vi "onHttpPatch (Buffer).vi"(8 "error in":errorcluster, 10 "httpRequest":refnum<class "httpRequest.lvclass">, 11 "http-method in":refnum<class "HttpClient.Basic.lvclass">) -> (0 "error out":errorcluster, 2 "httpResponse":refnum<class "httpResponse.lvclass">, 3 "http-method out":refnum<class "HttpClient.Basic.lvclass">)   [LabVIEW 2020, in "httpClient.lvlib" / "HttpClient.Basic.lvclass"]
uses:
  HttpClient.Basic.lvclass
  HttpClient.Basic.lvclass/HttpClient.Basic.ctl
  httpResponse/httpResponse.lvclass
  httpRequest/httpRequest.lvclass
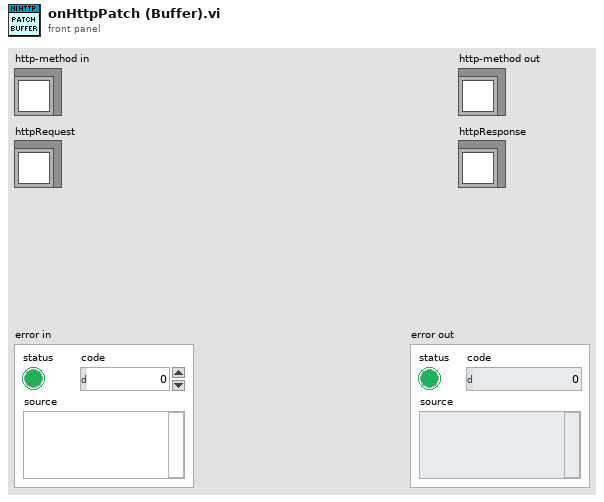
[diagram p1: front panel]
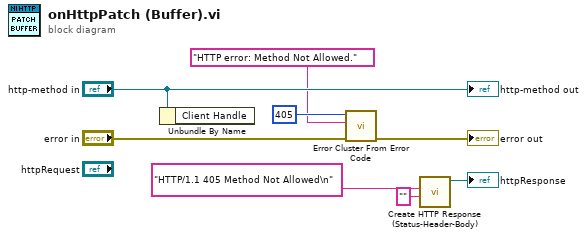
[diagram p0: block diagram]
diagram:
  n1 = Unbundle By Name("http-method in") -> ()  [unwired: 1 out]
  n2 = call <vilib>:"Error Cluster From Error Code.vi"("error in (no error)"="error in", "error message (\"\")"="HTTP error: Method Not Allowed.", "error code (0)"=405) -> ("error out"=→"error out":errorcluster)  [unwired: 6 in]
  n3 = call "Create HTTP Response (Status-Header-Body).vi"("body"="", "Headers w/ status line(s)"="HTTP/1.1 405 Method Not Allowed\n") -> ("httpResponse out"=→"httpResponse":refnum<class "httpResponse.lvclass">)  [unwired: 8 in, 1 out]
  "http-method out" <- "http-method in"
